vi "manual_control.vi"(0 "Elements+Rates":cluster{"Elements":u16[], "Rates":sgl[]}) -> ()   [LabVIEW 2012]
uses:
  elements.gbl
  number_of_sources.gbl
panel:
  in  "shutdown all":bool
  in  "close":bool
  out "Cluster references":refnum<vi>[][](array[refnum])
  in  "Frame":T1={"Element 1"={"Power (%)"=0.0, "Rate (Å/s)"=0.0, "Gain (Å/s/%)"=0.0, "Set gain"=FALSE, "Manual"=FALSE, "shutdown"=FALSE, "Plot range (min)"=10.0, "Rate graph"=[]}, "Element 2"={"Power (%)"=0.0, "Rate (Å/s)"=0.0, "Gain (Å/s/%)"=0.0, "Set gain"=FALSE, "Manual"=FALSE, "shutdown"=FALSE, "Plot range (min)"=10.0, "Rate graph"=[]}, "Element 3"={"Power (%)"=0.0, "Rate (Å/s)"=0.0, "Gain (Å/s/%)"=0.0, "Set gain"=FALSE, "Manual"=FALSE, "shutdown"=FALSE, "Plot range (min)"=10.0, "Rate graph"=[]}, "Element 4"={"Power (%)"=0.0, "Rate (Å/s)"=0.0, "Gain (Å/s/%)"=0.0, "Set gain"=FALSE, "Manual"=FALSE, "shutdown"=FALSE, "Plot range (min)"=10.0, "Rate graph"=[]}} {"Element 4"."Plot range (min)" min=0.025 step=1.0; "Element 4"."Rate (Å/s)" format="%#.2f"; "Element 4"."Power (%)" min=0 max=90 step=0.1 format="%.2f"; "Element 4"."Gain (Å/s/%)" format="%.1f"; "Element 3"."Plot range (min)" min=0.025 step=1.0; "Element 3"."Rate (Å/s)" format="%#.2f"; "Element 3"."Power (%)" min=0 max=90 step=0.1 format="%.2f"; "Element 3"."Gain (Å/s/%)" format="%.1f"; "Element 2"."Plot range (min)" min=0.025 step=1.0; "Element 2"."Rate (Å/s)" format="%#.2f"; "Element 2"."Power (%)" min=0 max=90 step=0.1 format="%.2f"; "Element 2"."Gain (Å/s/%)" format="%.1f"; "Element 1"."Plot range (min)" min=0.025 step=1.0; "Element 1"."Rate (Å/s)" format="%#.2f"; "Element 1"."Power (%)" min=0 max=90 step=0.1 format="%.2f"; "Element 1"."Gain (Å/s/%)" format="%.1f"}
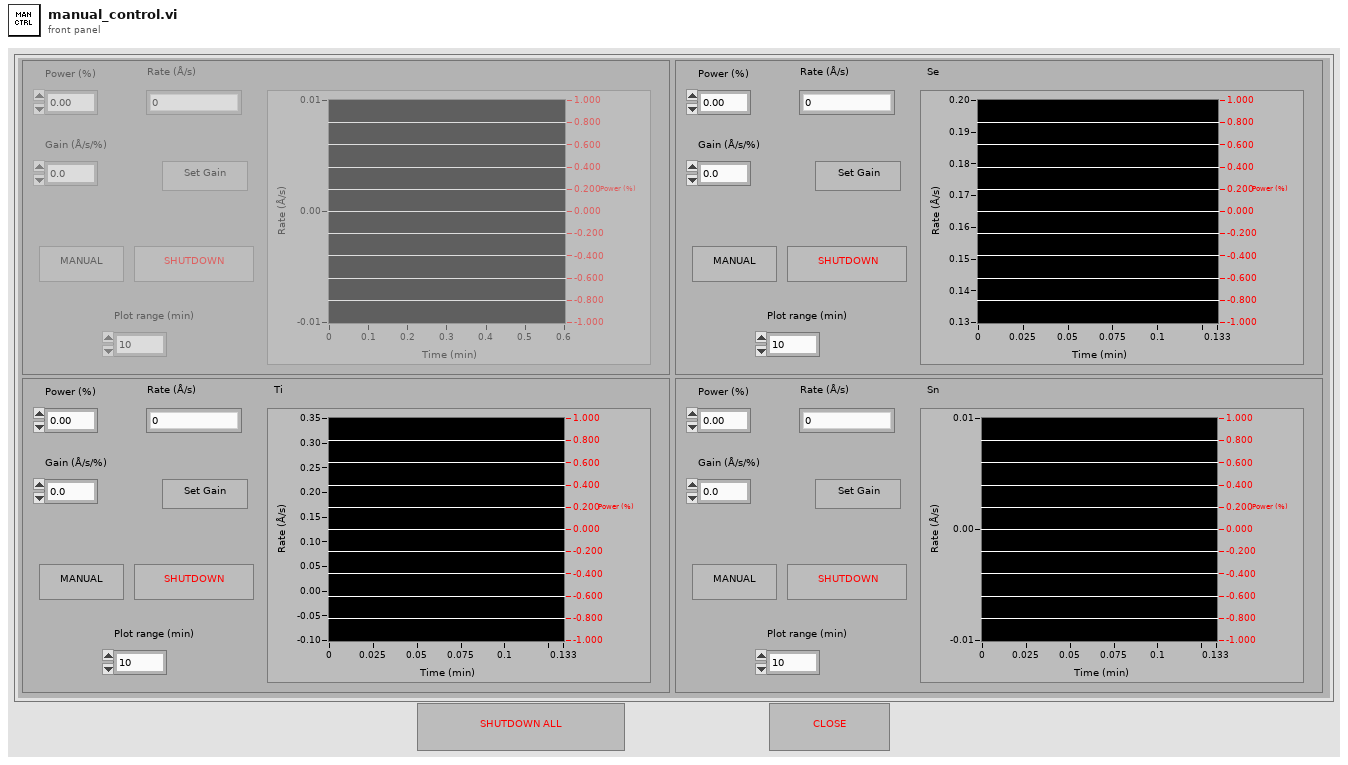
[diagram p1: front panel]
types:
  T1 = cluster{"Element 1":cluster{"Power (%)":sgl, "Rate (Å/s)":sgl, "Gain (Å/s/%)":sgl, "Set gain":bool, "Manual":bool, "shutdown":bool, "Plot range (min)":dbl, "Rate graph":cluster{cluster{sgl, sgl}[]}[]}, "Element 2":cluster{"Power (%)":sgl, "Rate (Å/s)":sgl, "Gain (Å/s/%)":sgl, "Set gain":bool, "Manual":bool, "shutdown":bool, "Plot range (min)":dbl, "Rate graph":cluster{cluster{sgl, sgl}[]}[]}, "Element 3":cluster{"Power (%)":sgl, "Rate (Å/s)":sgl, "Gain (Å/s/%)":sgl, "Set gain":bool, "Manual":bool, "shutdown":bool, "Plot range (min)":dbl, "Rate graph":cluster{cluster{sgl, sgl}[]}[]}, "Element 4":cluster{"Power (%)":sgl, "Rate (Å/s)":sgl, "Gain (Å/s/%)":sgl, "Set gain":bool, "Manual":bool, "shutdown":bool, "Plot range (min)":dbl, "Rate graph":cluster{cluster{sgl, sgl}[]}[]}}
  T2 = enum8{"Enabled", "Disabled", "Disabled and Grayed Out"}
  T3 = cluster{"Element 1":cluster{"Power (%)":bool, "Rate (Å/s)":bool, "Gain (Å/s/%)":bool, "Set gain":bool, "Manual":bool, "shutdown":bool, "Plot range (min)":bool, "Rate graph":cluster{cluster{bool, bool}[]}[]}, "Element 2":cluster{"Power (%)":bool, "Rate (Å/s)":bool, "Gain (Å/s/%)":bool, "Set gain":bool, "Manual":bool, "shutdown":bool, "Plot range (min)":bool, "Rate graph":cluster{cluster{bool, bool}[]}[]}, "Element 3":cluster{"Power (%)":bool, "Rate (Å/s)":bool, "Gain (Å/s/%)":bool, "Set gain":bool, "Manual":bool, "shutdown":bool, "Plot range (min)":bool, "Rate graph":cluster{cluster{bool, bool}[]}[]}, "Element 4":cluster{"Power (%)":bool, "Rate (Å/s)":bool, "Gain (Å/s/%)":bool, "Set gain":bool, "Manual":bool, "shutdown":bool, "Plot range (min)":bool, "Rate graph":cluster{cluster{bool, bool}[]}[]}}
  T4 = cluster{"Power (%)":bool, "Rate (Å/s)":bool, "Gain (Å/s/%)":bool, "Set gain":bool, "Manual":bool, "shutdown":bool, "Plot range (min)":bool, "Rate graph":cluster{cluster{bool, bool}[]}[]}[]
  T5 = cluster{"Power (%)":bool, "Set gain":bool, "Manual":bool, "shutdown":bool}
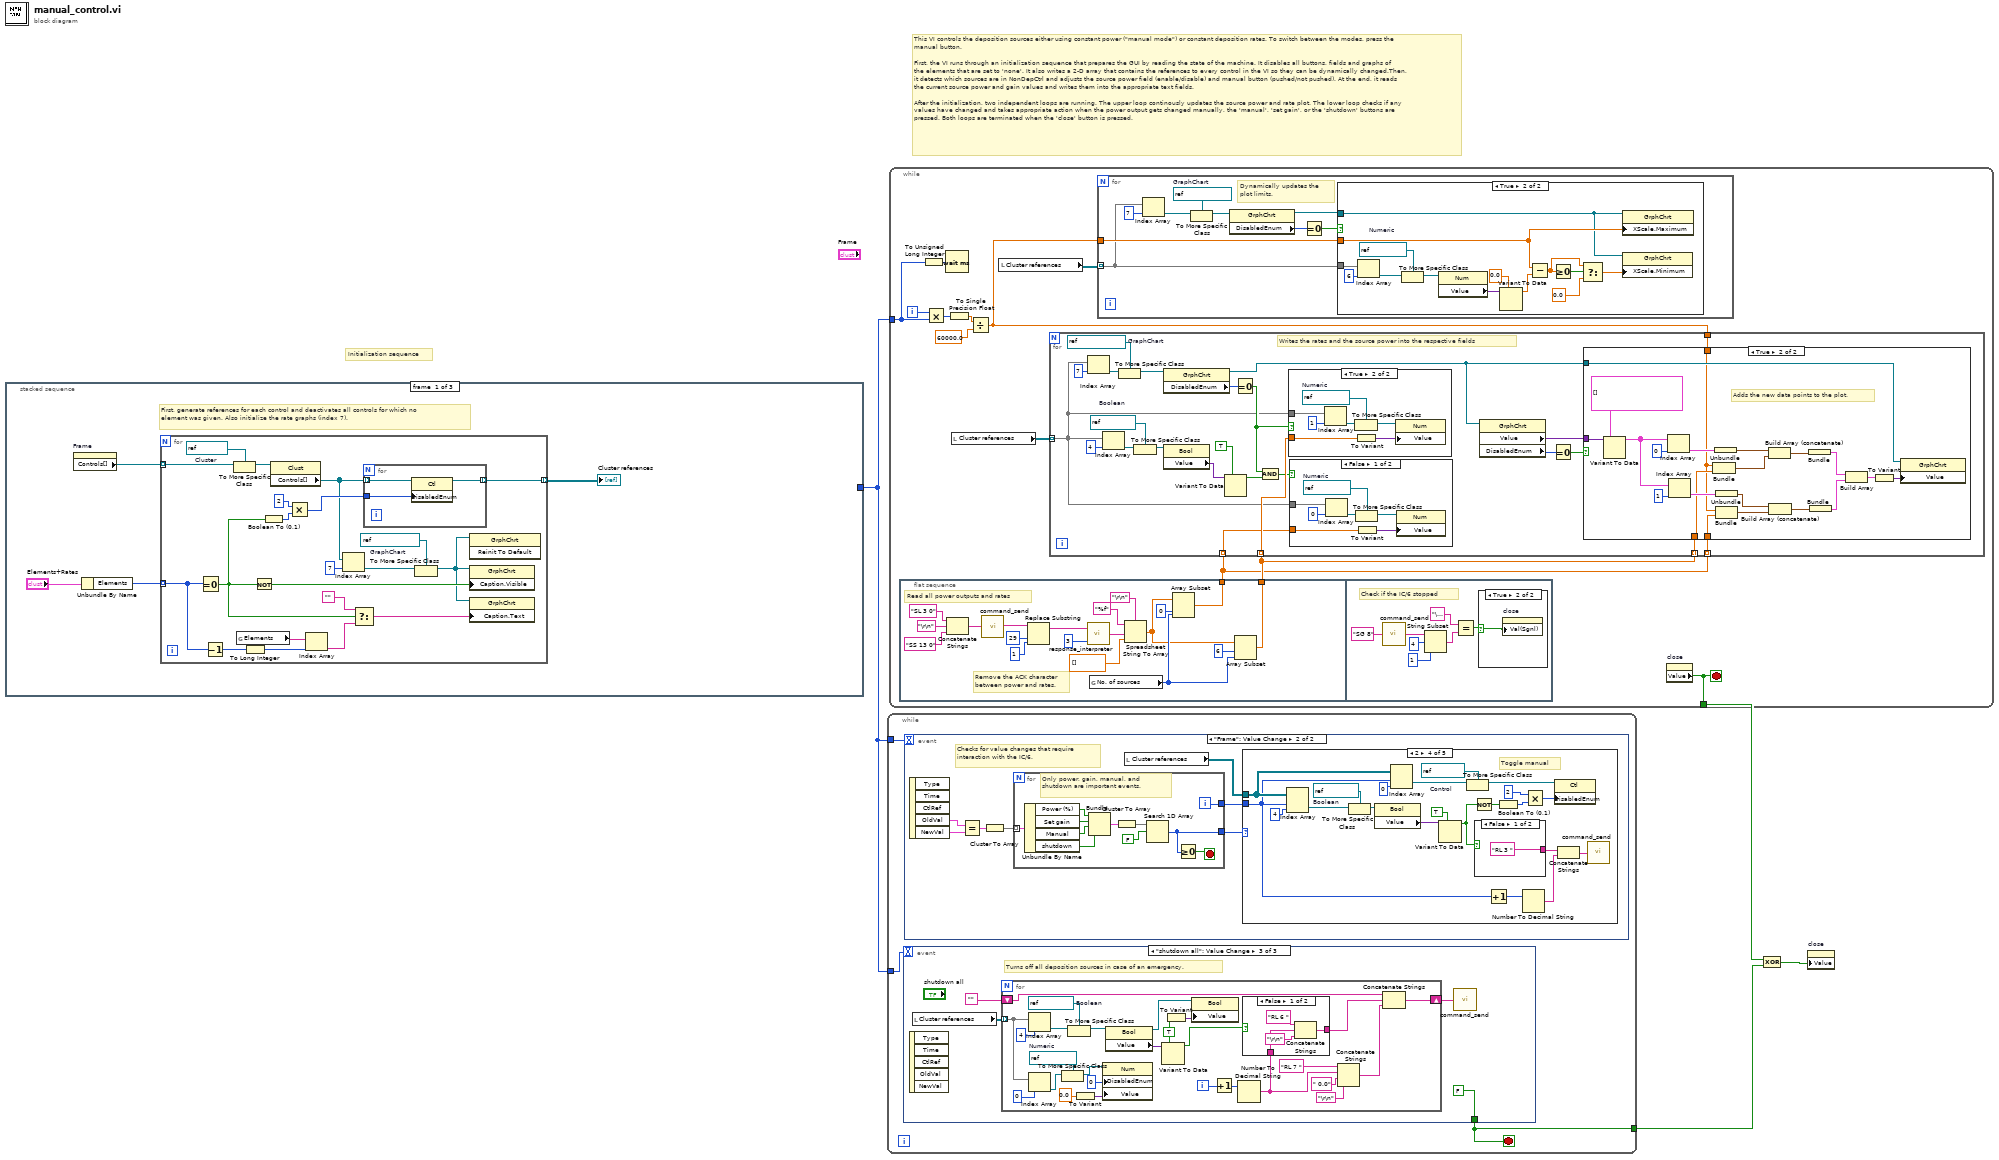
[diagram p0: block diagram]
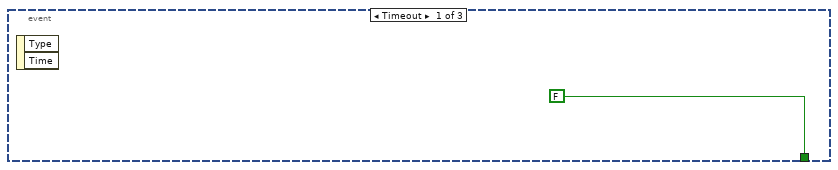
[diagram p2: hidden frame]
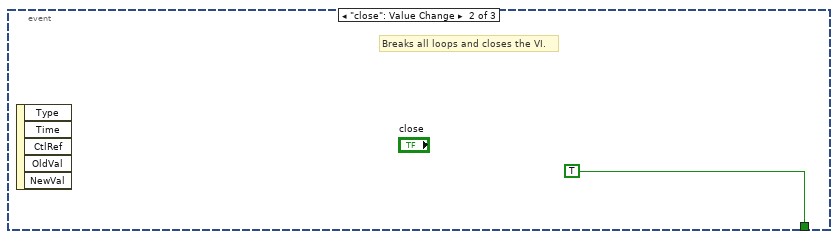
[diagram p3: hidden frame]
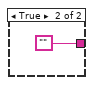
[diagram p4: hidden frame]
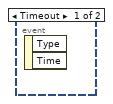
[diagram p5: hidden frame]
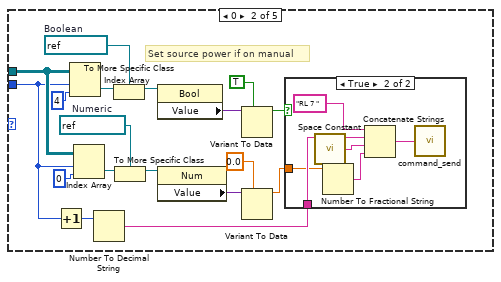
[diagram p7: hidden frame]
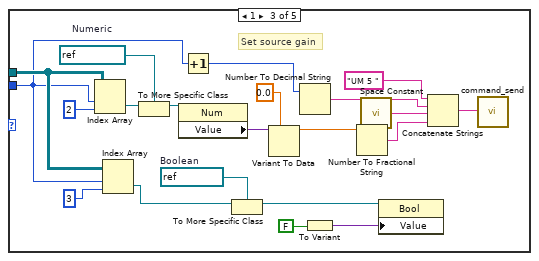
[diagram p9: hidden frame]
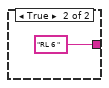
[diagram p10: hidden frame]
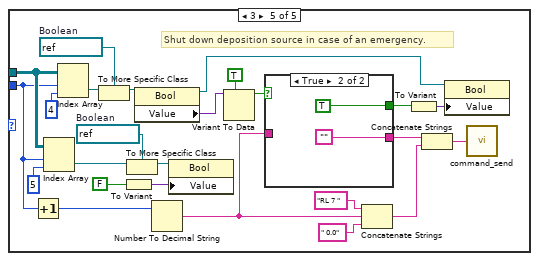
[diagram p11: hidden frame]
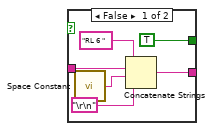
[diagram p12: hidden frame]
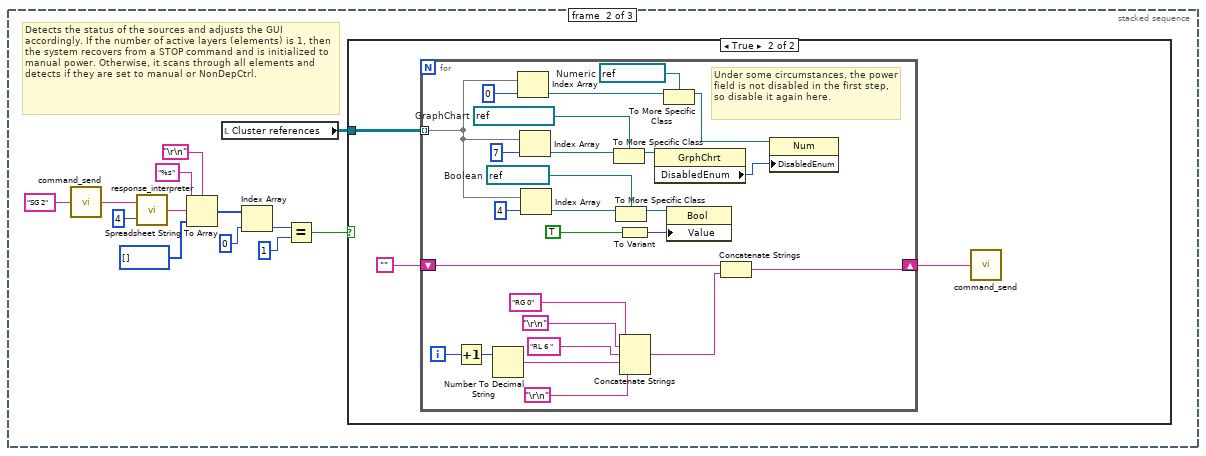
[diagram p18: hidden frame]
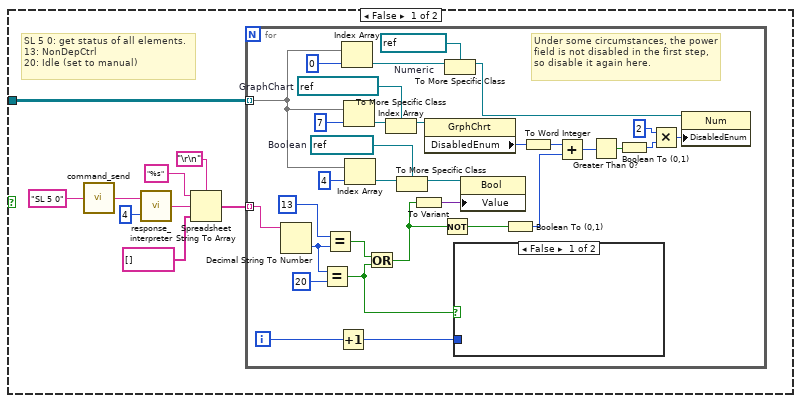
[diagram p19: hidden frame]
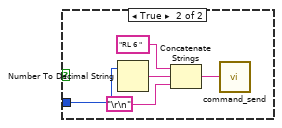
[diagram p20: hidden frame]
diagram:
  # "This VI controls the deposition sources either using constant power (\"manual mode\") or constant deposition rates. To switch between the modes, press the manual button.\n\nFirst, the VI runs through an initialization sequence that prepares the GUI by reading the state of the machine. It disables all buttons, fields and graphs of the elements that are set to 'none'. It also writes a 2-D array that contains the references to every control in the VI so they can be dynamically changed.Then, it detects which sources are in NonDepCtrl and adjusts the source power field (enable/disable) and manual button (pushed/not pushed). At the end, it reads the current source power and gain values and writes them into the appropriate text fields.\n\nAfter the initialization, two independent loops are running. The upper loop continously updates the source power and rate plot. The lower loop checks if any values have changed and takes appropriate action when the power output gets changed manually, the 'manual', 'set gain', or the 'shutdown' buttons are pressed. Both loops are terminated when the 'close' button is pressed."
  # "Initialization sequence"
  n1 = stacked-sequence {
    tunnel: [_ _ 500] -> w4
    frame #0 {
      # "First, generate references for each control and deactivates all controls for which no element was given. Also initialize the rate graphs (index 7)."
      n2 = property on="Frame" class="Clust (strict)"() -> ("Controls[]"=w6:refnum<vi>[])  [unwired: 2 in, 2 out]
      n3 = Unbundle By Name("Elements+Rates") -> ("Elements"=w7:u16[])
      n4 = for {
        tunnel: w7 -> [w13] mode=indexing
        tunnel: w6 -> [w24] mode=indexing
        tunnel: [w23] -> w5 mode=indexing
        w11 = refnum<vi> refnum  # GraphChart
        w26 = refnum<vi> refnum  # Cluster
        n5 = Equal To 0?(x=w13) -> (x = 0?=w15:bool)
        n6 = Decrement(x=w13) -> (x-1=w14:u16)
        n7 = To More Specific Class(target class=w26, reference=w24) -> (specific class reference=w25:refnum<vi>)  [unwired: 1 in, 1 out]
        n8 = global read "elements.gbl" "Elements"() -> (w28:string[])
        n9 = To Long Integer(number=w14) -> (32bit integer=w9:i32)
        n10 = Not(x=w15) -> (.not. x?=w18:bool)
        n11 = Boolean To (0,1)(Boolean=w15) -> (0, 1=w21:i16)
        n12 = property class="Clust"(reference=w25) -> ("Controls[]"=w19:refnum<vi>[])  [unwired: 1 in, 2 out]
        n13 = Multiply(x=i16 2, y=w21) -> (x*y=w20:i16)
        n14 = Index Array(array=w28, index=w9) -> (element=w16:string)
        n15 = Index Array(array=w19, index=7) -> (element=w12:refnum<vi>)
        n16 = Select(t="", s=w15, f=w16) -> (s? t:f=w27:string)
        n17 = for {
          tunnel: w19 -> [w32] mode=indexing
          tunnel: [w31] -> w23 mode=indexing
          tunnel: w20 -> [w30]
          n18 = property class="Ctl"(reference=w32, "DisabledEnum"=w30) -> (reference out=w31:refnum<vi>)  [unwired: 1 in, 1 out]
        }
        n19 = To More Specific Class(target class=w11, reference=w12) -> (specific class reference=w10:refnum<vi>)  [unwired: 1 in, 1 out]
        n20 = invoke class="GrphChrt" method="Reinit To Default"(reference=w10) -> ()  [unwired: 2 in, 3 out]
        n21 = property class="GrphChrt"(reference=w10, "Caption.Visible"=w18) -> ()  [unwired: 1 in, 2 out]
        n22 = property class="GrphChrt"(reference=w10, "Caption.Text"=w27) -> ()  [unwired: 1 in, 2 out]
      }
      "Cluster references" <- w5
    }
    frame #1 {
      # "Detects the status of the sources and adjusts the GUI accordingly. If the number of active layers (elements) is 1, then the system recovers from a STOP command and is initialized to manual power. Otherwise, it scans through all elements and detects if they are set to manual or NonDepCtrl."
      n23 = call "command_send.vi"("Commands"="SG 2") -> ("Response"=w43:string)
      n24 = call "response_interpreter.vi"("Response type"=u16 4, "Response hex"=w43) -> ("Response (readable)"=w42:string)
      n25 = Spreadsheet String To Array(delimiter (Tab)="\r\n", format string="%s", spreadsheet string=w42, array type (2D Dbl)=i32[] []) -> (array=w39:i32[])
      n26 = local read "Cluster references"() -> (w33:refnum<vi>[][])
      n27 = Index Array(array=w39, index=0) -> (element=w36:i32)
      n28 = Equal?(x=w36, y=1) -> (x = y?=w34:bool)
      n29 = case shown="True" w34 {
        tunnel: w33 -> [w46 w94]
        frame False {
          # "SL 5 0: get status of all elements.\n13: NonDepCtrl\n20: Idle (set to manual)"
          n30 = call "command_send.vi"("Commands"="SL 5 0") -> ("Response"=w53:string)
          n31 = call "response_interpreter.vi"("Response type"=u16 4, "Response hex"=w53) -> ("Response (readable)"=w49:string)
          n32 = Spreadsheet String To Array(delimiter (Tab)="\r\n", format string="%s", spreadsheet string=w49, array type (2D Dbl)=string[] []) -> (array=w47:string[])
          n33 = for {
            tunnel: w47 -> [w69] mode=indexing
            tunnel: w46 -> [w73] mode=indexing
            i -> [w65]
            w75 = refnum<vi> refnum  # Numeric
            w80 = refnum<vi> refnum  # Boolean
            w83 = refnum<vi> refnum  # GraphChart
            # "Under some circumstances, the power field is not disabled in the first step, so disable it again here."
            n34 = Decimal String To Number(string=w69) -> (number=w71:i32)  [unwired: 2 in, 1 out]
            n35 = Equal?(x=w71, y=20) -> (x = y?=w67:bool)
            n36 = Equal?(x=13, y=w71) -> (x = y?=w68:bool)
            n37 = Increment(x=w65) -> (x+1=w66:i32)
            n38 = Index Array(array=w73, index=0) -> (element=w76:refnum<vi>)
            n39 = Index Array(array=w73, index=7) -> (element=w85:refnum<vi>)
            n40 = Index Array(array=w73, index=4) -> (element=w81:refnum<vi>)
            n41 = Or(x=w68, y=w67) -> (x .or. y?=w64:bool)
            n42 = To More Specific Class(target class=w83, reference=w85) -> (specific class reference=w84:refnum<vi>)  [unwired: 1 in, 1 out]
            n43 = To More Specific Class(target class=w80, reference=w81) -> (specific class reference=w79:refnum<vi>)  [unwired: 1 in, 1 out]
            n44 = To Variant(anything=w64) -> (Variant=w78:variant)
            n45 = property class="GrphChrt"(reference=w84) -> ("DisabledEnum"=w57:T2)  [unwired: 1 in, 2 out]
            n46 = Not(x=w64) -> (.not. x?=w59:bool)
            n47 = To More Specific Class(target class=w75, reference=w76) -> (specific class reference=w74:refnum<vi>)  [unwired: 1 in, 1 out]
            n48 = case shown="False" w67 {
              tunnel: w66 -> [_ w87]
              frame False {
              }
              frame True {
                n49 = Number To Decimal String(number=w87) -> (decimal integer string=w89:string)  [unwired: 1 in]
                n50 = Concatenate Strings("RL 6 ", w89, "\r\n") -> (w88:string)
                n51 = call "command_send.vi"("Commands"=w88) -> ()  [unwired: 1 out]
              }
            }
            n52 = property class="Bool"(reference=w79, "Value"=w78) -> ()  [unwired: 1 in, 2 out]
            n53 = Boolean To (0,1)(Boolean=w59) -> (0, 1=w56:i16)
            n54 = To Word Integer(number=w57) -> (16bit integer=w55:i16)
            n55 = Add(x=w55, y=w56) -> (x+y=w58:i16)
            n56 = Greater Than 0?(x=w58) -> (x > 0?=w60:bool)
            n57 = Boolean To (0,1)(Boolean=w60) -> (0, 1=w61:i16)
            n58 = Multiply(x=i16 2, y=w61) -> (x*y=w63:i16)
            n59 = property class="Num"(reference=w74, "DisabledEnum"=w63) -> ()  [unwired: 1 in, 2 out]
          }
        }
        frame True {
          n60 = for {
            tunnel: w94 -> [w100] mode=indexing
            shift-right: [w101] -> w92
            shift-left: "" -> [w102]
            i -> [w104]
            w97 = refnum<vi> refnum  # Numeric
            w114 = refnum<vi> refnum  # Boolean
            w117 = refnum<vi> refnum  # GraphChart
            # "Under some circumstances, the power field is not disabled in the first step, so disable it again here."
            n61 = Increment(x=w104) -> (x+1=w105:i32)
            n62 = Number To Decimal String(number=w105) -> (decimal integer string=w110:string)  [unwired: 1 in]
            n63 = Index Array(array=w100, index=0) -> (element=w98:refnum<vi>)
            n64 = Index Array(array=w100, index=7) -> (element=w119:refnum<vi>)
            n65 = Index Array(array=w100, index=4) -> (element=w115:refnum<vi>)
            n66 = To More Specific Class(target class=w117, reference=w119) -> (specific class reference=w118:refnum<vi>)  [unwired: 1 in, 1 out]
            n67 = To More Specific Class(target class=w114, reference=w115) -> (specific class reference=w113:refnum<vi>)  [unwired: 1 in, 1 out]
            n68 = To Variant(anything=TRUE) -> (Variant=w111:variant)
            n69 = Concatenate Strings("RG 0", "\r\n", "RL 6 ", w110, "\r\n") -> (w103:string)
            n70 = property class="GrphChrt"(reference=w118) -> ("DisabledEnum"=w95:T2)  [unwired: 1 in, 2 out]
            n71 = To More Specific Class(target class=w97, reference=w98) -> (specific class reference=w96:refnum<vi>)  [unwired: 1 in, 1 out]
            n72 = property class="Bool"(reference=w113, "Value"=w111) -> ()  [unwired: 1 in, 2 out]
            n73 = Concatenate Strings(w102, w103) -> (w101:string)
            n74 = property class="Num"(reference=w96, "DisabledEnum"=w95) -> ()  [unwired: 1 in, 2 out]
          }
          n75 = call "command_send.vi"("Commands"=w92) -> ()  [unwired: 1 out]
        }
      }
    }
    frame #2 {
      # "At last, read the current power output (SL 3) and the gain (QM 5) for each element, and write them into the appropriate fields."
      n76 = call "command_send.vi"("Commands"="SL 3 0") -> ("Response"=w129:string)
      n77 = local read "Cluster references"() -> (w122:refnum<vi>[][])
      n78 = call "response_interpreter.vi"("Response type"=u16 3, "Response hex"=w129) -> ("Response (readable)"=w125:string)
      n79 = Spreadsheet String To Array(delimiter (Tab)="\r\n", format string="%f", spreadsheet string=w125, array type (2D Dbl)=sgl[] []) -> (array=w123:sgl[])
      n80 = for {
        tunnel: w123 -> [w138] mode=indexing
        tunnel: w122 -> [w137] mode=indexing
        i -> [w151]
        w139 = refnum<vi> refnum  # Numeric
        w141 = refnum<vi> refnum  # Numeric
        n81 = Increment(x=w151) -> (x+1=w150:i32)
        n82 = Number To Decimal String(number=w150) -> (decimal integer string=w149:string)  [unwired: 1 in]
        n83 = Concatenate Strings("QM 5 ", w149) -> (w148:string)
        n84 = call "command_send.vi"("Commands"=w148) -> ("Response"=w147:string)
        n85 = Index Array(array=w137, index=0) -> (element=w143:refnum<vi>)
        n86 = Index Array(array=w137, index=2) -> (element=w136:refnum<vi>)
        n87 = call "response_interpreter.vi"("Response type"=u16 3, "Response hex"=w147) -> ("Response (readable)"=w132:string)
        n88 = To Variant(anything=w138) -> (Variant=w140:variant)
        n89 = To More Specific Class(target class=w141, reference=w143) -> (specific class reference=w142:refnum<vi>)  [unwired: 1 in, 1 out]
        n90 = To More Specific Class(target class=w139, reference=w136) -> (specific class reference=w135:refnum<vi>)  [unwired: 1 in, 1 out]
        n91 = Fract/Exp String To Number(string=w132, default (0 dbl)=sgl 0.0) -> (number=w131:sgl)  [unwired: 2 in, 1 out]
        n92 = property class="Num"(reference=w142, "Value"=w140) -> ()  [unwired: 1 in, 2 out]
        n93 = To Variant(anything=w131) -> (Variant=w134:variant)
        n94 = property class="Num"(reference=w135, "Value"=w134) -> ()  [unwired: 1 in, 2 out]
      }
    }
  }
  n95 = while {
    tunnel: w4 -> [w155]
    tunnel: w4 -> [w154]
    tunnel: [w153] -> w3
    stop <- w153 stop-if-true
    n96 = event shown="[2] \"shutdown all\": Value Change" {
      selector: _ -> [_ _ _]
      dyn-events: _ -> [_ _ _]
      timeout: w154 -> [_ _ _]
      tunnel: [FALSE TRUE FALSE] -> w153
      event Timeout {
        n97 = event-data() -> ()  [unwired: 1 in, 2 out]
      }
      event "close": Value Change {
        # "Breaks all loops and closes the VI."
        n98 = event-data() -> ()  [unwired: 1 in, 5 out]
      }
      event "shutdown all": Value Change {
        # "Turns off all deposition sources in case of an emergency."
        n99 = event-data() -> ()  [unwired: 1 in, 5 out]
        n100 = local read "Cluster references"() -> (w160:refnum<vi>[][])
        n101 = for {
          tunnel: w160 -> [w175] mode=indexing
          shift-right: [w187] -> w158
          shift-left: "" -> [w188]
          i -> [w179]
          w169 = TRUE
          w167 = refnum<vi> refnum  # Numeric
          w177 = refnum<vi> refnum  # Boolean
          n102 = Index Array(array=w175, index=4) -> (element=w178:refnum<vi>)
          n103 = Index Array(array=w175, index=0) -> (element=w166:refnum<vi>)
          n104 = To More Specific Class(target class=w167, reference=w166) -> (specific class reference=w165:refnum<vi>)  [unwired: 1 in, 1 out]
          n105 = To More Specific Class(target class=w177, reference=w178) -> (specific class reference=w173:refnum<vi>)  [unwired: 1 in, 1 out]
          n106 = To Variant(anything=0.0) -> (Variant=w163:variant)
          n107 = property class="Num"(reference=w165, "DisabledEnum"=0, "Value"=w163) -> ()  [unwired: 1 in, 2 out]
          n108 = property class="Bool"(reference=w173) -> (reference out=w168:refnum<vi>, "Value"=w172:variant)  [unwired: 1 in, 1 out]
          n109 = Variant To Data(type=w169, Variant=w172) -> (data=w171:bool)  [unwired: 1 in, 1 out]
          n110 = To Variant(anything=w169) -> (Variant=w170:variant)
          n111 = property class="Bool"(reference=w168, "Value"=w170) -> ()  [unwired: 1 in, 2 out]
          n112 = Increment(x=w179) -> (x+1=w182:i32)
          n113 = Number To Decimal String(number=w182) -> (decimal integer string=w180:string)  [unwired: 1 in]
          n114 = case shown="False" w171 {
            tunnel: [w190 ""] -> w186
            tunnel: w180 -> [w189 _]
            frame False {
              n115 = Concatenate Strings("RL 6 ", w189, "\r\n") -> (w190:string)
            }
            frame True {
            }
          }
          n116 = Concatenate Strings("RL 7 ", w180, " 0.0", "\r\n") -> (w181:string)
          n117 = Concatenate Strings(w188, w186, w181) -> (w187:string)
        }
        n118 = call "command_send.vi"("Commands"=w158) -> ()  [unwired: 1 out]
      }
    }
    n119 = event shown="[1] \"Frame\": Value Change" {
      selector: _ -> [_ _]
      dyn-events: _ -> [_ _]
      timeout: w155 -> [_ _]
      event Timeout {
        n120 = event-data() -> ()  [unwired: 1 in, 2 out]
      }
      event "Frame": Value Change {
        # "Checks for value changes that require interaction with the IC/6."
        n121 = event-data() -> ("OldVal"=w200:T1, "NewVal"=w199:T1)  [unwired: 1 in, 3 out]
        n122 = Equal?(x=w200, y=w199) -> (x = y?=w198:T3)
        n123 = Cluster To Array(cluster=w198) -> (array=w197:T4)
        n124 = for {
          tunnel: w197 -> [w312] mode=indexing
          tunnel: [w304] -> w196
          tunnel: [w302] -> w194
          i -> [w302]
          stop <- w305 stop-if-true
          # "Only power, gain, manual, and shutdown are important events."
          n125 = Unbundle By Name(w312) -> ("Power (%)"=w311:bool, "Set gain"=w310:bool, "Manual"=w309:bool, "shutdown"=w308:bool)
          n126 = Bundle("Power (%)"=w311, "Set gain"=w310, "Manual"=w309, "shutdown"=w308) -> (w307:T5)  [unwired: 1 in]
          n127 = Cluster To Array(cluster=w307) -> (array=w306:bool[])
          n128 = Search 1D Array(1D array=w306, element=FALSE) -> (index of element=w304:i32)  [unwired: 1 in]
          n129 = Greater Or Equal To 0?(x=w304) -> (x >= 0?=w305:bool)
        }
        n130 = local read "Cluster references"() -> (w195:refnum<vi>[][])
        n131 = case shown="2" w196 {
          tunnel: w195 -> [_ w214 w232 w248 w271]
          tunnel: w194 -> [_ w203 w231 w247 w270]
          frame -1, Default {
          }
          frame 0 {
            w218 = refnum<vi> refnum  # Numeric
            w217 = refnum<vi> refnum  # Boolean
            # "Set source power if on manual"
            n132 = Increment(x=w203) -> (x+1=w202:i32)
            n133 = Index Array(array=w214, index (row)=w203, index (col)=4) -> (element=w216:refnum<vi>)
            n134 = Index Array(array=w214, index (row)=w203, index (col)=0) -> (element=w215:refnum<vi>)
            n135 = Number To Decimal String(number=w202) -> (decimal integer string=w201:string)  [unwired: 1 in]
            n136 = To More Specific Class(target class=w217, reference=w216) -> (specific class reference=w211:refnum<vi>)  [unwired: 1 in, 1 out]
            n137 = To More Specific Class(target class=w218, reference=w215) -> (specific class reference=w210:refnum<vi>)  [unwired: 1 in, 1 out]
            n138 = property class="Bool"(reference=w211) -> ("Value"=w209:variant)  [unwired: 1 in, 2 out]
            n139 = property class="Num"(reference=w210) -> ("Value"=w208:variant)  [unwired: 1 in, 2 out]
            n140 = Variant To Data(type=TRUE, Variant=w209) -> (data=w205:bool)  [unwired: 1 in, 1 out]
            n141 = Variant To Data(type=sgl 0.0, Variant=w208) -> (data=w204:sgl)  [unwired: 1 in, 1 out]
            n142 = case shown="True" w205 {
              tunnel: w204 -> [_ w219]
              tunnel: w201 -> [_ w220]
              frame False {
              }
              frame True {
                n143 = call <vilib>:"Space Constant.vi"() -> ("String"=w221:string)
                n144 = Number To Fractional String(number=w219) -> (F-format string=w224:string)  [unwired: 3 in]
                n145 = Concatenate Strings("RL 7 ", w220, w221, w224) -> (w223:string)
                n146 = call "command_send.vi"("Commands"=w223) -> ()  [unwired: 1 out]
              }
            }
          }
          frame 1 {
            w226 = refnum<vi> refnum  # Boolean
            w242 = refnum<vi> refnum  # Numeric
            # "Set source gain"
            n147 = Index Array(array=w232, index (row)=w231, index (col)=2) -> (element=w241:refnum<vi>)
            n148 = Index Array(array=w232, index (row)=w231, index (col)=3) -> (element=w229:refnum<vi>)
            n149 = To More Specific Class(target class=w242, reference=w241) -> (specific class reference=w240:refnum<vi>)  [unwired: 1 in, 1 out]
            n150 = property class="Num"(reference=w240) -> ("Value"=w239:variant)  [unwired: 1 in, 2 out]
            n151 = Increment(x=w231) -> (x+1=w233:i32)
            n152 = To More Specific Class(target class=w226, reference=w229) -> (specific class reference=w228:refnum<vi>)  [unwired: 1 in, 1 out]
            n153 = Variant To Data(type=sgl 0.0, Variant=w239) -> (data=w237:sgl)  [unwired: 1 in, 1 out]
            n154 = Number To Decimal String(number=w233) -> (decimal integer string=w234:string)  [unwired: 1 in]
            n155 = To Variant(anything=FALSE) -> (Variant=w225:variant)
            n156 = Number To Fractional String(number=w237) -> (F-format string=w245:string)  [unwired: 3 in]
            n157 = call <vilib>:"Space Constant.vi"() -> ("String"=w235:string)
            n158 = property class="Bool"(reference=w228, "Value"=w225) -> ()  [unwired: 1 in, 2 out]
            n159 = Concatenate Strings("UM 5 ", w234, w235, w245) -> (w244:string)
            n160 = call "command_send.vi"("Commands"=w244) -> ()  [unwired: 1 out]
          }
          frame 2 {
            w250 = refnum<vi> refnum  # Control
            w264 = refnum<vi> refnum  # Boolean
            # "Toggle manual"
            n161 = Index Array(array=w248, index (row)=w247, index (col)=4) -> (element=w265:refnum<vi>)
            n162 = To More Specific Class(target class=w264, reference=w265) -> (specific class reference=w263:refnum<vi>)  [unwired: 1 in, 1 out]
            n163 = property class="Bool"(reference=w263) -> ("Value"=w262:variant)  [unwired: 1 in, 2 out]
            n164 = Index Array(array=w248, index (row)=w247, index (col)=0) -> (element=w252:refnum<vi>)
            n165 = Variant To Data(type=TRUE, Variant=w262) -> (data=w257:bool)  [unwired: 1 in, 1 out]
            n166 = To More Specific Class(target class=w250, reference=w252) -> (specific class reference=w251:refnum<vi>)  [unwired: 1 in, 1 out]
            n167 = Not(x=w257) -> (.not. x?=w258:bool)
            n168 = case shown="False" w257 {
              tunnel: ["RL 3 " "RL 6 "] -> w259
              frame False {
              }
              frame True {
              }
            }
            n169 = Increment(x=w247) -> (x+1=w260:i32)
            n170 = Boolean To (0,1)(Boolean=w258) -> (0, 1=w256:i16)
            n171 = Number To Decimal String(number=w260) -> (decimal integer string=w255:string)  [unwired: 1 in]
            n172 = Multiply(x=i16 2, y=w256) -> (x*y=w249:i16)
            n173 = property class="Ctl"(reference=w251, "DisabledEnum"=w249) -> ()  [unwired: 1 in, 2 out]
            n174 = Concatenate Strings(w259, w255) -> (w246:string)
            n175 = call "command_send.vi"("Commands"=w246) -> ()  [unwired: 1 out]
          }
          frame 3 {
            w276 = refnum<vi> refnum  # Boolean
            w281 = refnum<vi> refnum  # Boolean
            # "Shut down deposition source in case of an emergency."
            n176 = Increment(x=w270) -> (x+1=w293:i32)
            n177 = Index Array(array=w271, index (row)=w270, index (col)=5) -> (element=w272:refnum<vi>)
            n178 = Index Array(array=w271, index (row)=w270, index (col)=4) -> (element=w282:refnum<vi>)
            n179 = To More Specific Class(target class=w281, reference=w282) -> (specific class reference=w280:refnum<vi>)  [unwired: 1 in, 1 out]
            n180 = To Variant(anything=FALSE) -> (Variant=w274:variant)
            n181 = To More Specific Class(target class=w276, reference=w272) -> (specific class reference=w275:refnum<vi>)  [unwired: 1 in, 1 out]
            n182 = property class="Bool"(reference=w280) -> (reference out=w278:refnum<vi>, "Value"=w279:variant)  [unwired: 1 in, 1 out]
            n183 = Number To Decimal String(number=w293) -> (decimal integer string=w290:string)  [unwired: 1 in]
            n184 = property class="Bool"(reference=w275, "Value"=w274) -> ()  [unwired: 1 in, 2 out]
            n185 = Variant To Data(type=TRUE, Variant=w279) -> (data=w285:bool)  [unwired: 1 in, 1 out]
            n186 = case shown="True" w285 {
              tunnel: [w299 ""] -> w289
              tunnel: w290 -> [w295 _]
              tunnel: [TRUE TRUE] -> w286
              frame False {
                n187 = call <vilib>:"Space Constant.vi"() -> ("String"=w296:string)
                n188 = Concatenate Strings("RL 6 ", w295, w296, "\r\n") -> (w299:string)
              }
              frame True {
              }
            }
            n189 = Concatenate Strings("RL 7 ", w290, " 0.0") -> (w288:string)
            n190 = To Variant(anything=w286) -> (Variant=w277:variant)
            n191 = Concatenate Strings(w289, w288) -> (w287:string)
            n192 = property class="Bool"(reference=w278, "Value"=w277) -> ()  [unwired: 1 in, 2 out]
            n193 = call "command_send.vi"("Commands"=w287) -> ()  [unwired: 1 out]
          }
        }
      }
    }
  }
  n194 = while {
    tunnel: w4 -> [w323]
    tunnel: [w317] -> w2
    i -> [w324]
    stop <- w317 stop-if-true
    n195 = flat-sequence {
      tunnel: [w415] -> w315
      tunnel: [w414] -> w316
      frame #0 {
        # "Remove the ACK character between power and rates."
        # "Read all power outputs and rates"
        n196 = Concatenate Strings("SL 3 0", "\r\n", "SS 13 0") -> (w420:string)
        n197 = call "command_send.vi"("Commands"=w420) -> ("Response"=w407:string)
        n198 = Replace Substring(2:1, 3:29, 5:w407) -> (1:w410:string)  [unwired: 1 in, 1 out]
        n199 = call "response_interpreter.vi"("Response type"=u16 3, "Response hex"=w410) -> ("Response (readable)"=w423:string)
        n200 = global read "number_of_sources.gbl" "No. of sources"() -> (w412:i32)
        n201 = Spreadsheet String To Array(delimiter (Tab)="\r\n", format string="%f", spreadsheet string=w423, array type (2D Dbl)=sgl[] []) -> (array=w411:sgl[])
        n202 = Array Subset(array=w411, index=0, length=w412) -> (w415:sgl[])
        n203 = Array Subset(array=w411, index=6, length=w412) -> (w414:sgl[])
      }
      frame #1 {
        # "Check if the IC/6 stopped"
        n204 = call "command_send.vi"("Commands"="SG 8") -> ("Response"=w431:string)
        n205 = String Subset(string=w431, offset (0)=4, length (rest)=1) -> (substring=w427:string)
        n206 = Equal?(x="\u0006", y=w427) -> (x = y?=w426:bool)
        n207 = case shown="True" w426 {
          selector: w426 -> [_ w433]
          frame False {
          }
          frame True {
            n208 = property on="close" class="Bool (strict)"("Val(Sgnl)"=w433) -> ()  [unwired: 2 in, 2 out]
          }
        }
      }
    }
    n209 = To Unsigned Long Integer(number=w323) -> (unsigned 32bit integer=w314:u32)
    n210 = Multiply(x=w324, y=w323) -> (x*y=w322:i32)
    n211 = Wait (ms)(milliseconds to wait=w314) -> ()  [unwired: 1 out]
    n212 = To Single Precision Float(number=w322) -> (single precision float=w313:sgl)
    n213 = local read "Cluster references"() -> (w319:refnum<vi>[][])
    n214 = Divide(x=w313, y=sgl 60000.0) -> (x/y=w318:sgl)
    n215 = local read "Cluster references"() -> (w320:refnum<vi>[][])
    n216 = for {
      tunnel: w319 -> [w330] mode=indexing
      tunnel: w315 -> [w329] mode=indexing
      tunnel: w316 -> [w332] mode=indexing
      tunnel: w318 -> [w328]
      tunnel: w315 -> [w327] mode=indexing
      tunnel: w316 -> [w326] mode=indexing
      w342 = refnum<vi> refnum  # Boolean
      w347 = refnum<vi> refnum  # GraphChart
      # "Writes the rates and the source power into the respective fields"
      n217 = Index Array(array=w330, index=7) -> (element=w346:refnum<vi>)
      n218 = Index Array(array=w330, index=4) -> (element=w341:refnum<vi>)
      n219 = To More Specific Class(target class=w347, reference=w346) -> (specific class reference=w337:refnum<vi>)  [unwired: 1 in, 1 out]
      n220 = To More Specific Class(target class=w342, reference=w341) -> (specific class reference=w340:refnum<vi>)  [unwired: 1 in, 1 out]
      n221 = property class="Bool"(reference=w340) -> ("Value"=w339:variant)  [unwired: 1 in, 2 out]
      n222 = property class="GrphChrt"(reference=w337) -> (reference out=w325:refnum<vi>, "DisabledEnum"=w345:T2)  [unwired: 1 in, 1 out]
      n223 = Variant To Data(type=TRUE, Variant=w339) -> (data=w338:bool)  [unwired: 1 in, 1 out]
      n224 = Equal To 0?(x=w345) -> (x = 0?=w333:bool)
      n225 = And(x=w333, y=w338) -> (x .and. y?=w331:bool)
      n226 = case shown="True" w333 {
        tunnel: w330 -> [_ w352]
        tunnel: w332 -> [_ w349]
        frame False {
        }
        frame True {
          w355 = refnum<vi> refnum  # Numeric
          n227 = Index Array(array=w352, index=1) -> (element=w354:refnum<vi>)
          n228 = To More Specific Class(target class=w355, reference=w354) -> (specific class reference=w351:refnum<vi>)  [unwired: 1 in, 1 out]
          n229 = To Variant(anything=w349) -> (Variant=w350:variant)
          n230 = property class="Num"(reference=w351, "Value"=w350) -> ()  [unwired: 1 in, 2 out]
        }
      }
      n231 = case shown="False" w331 {
        tunnel: w330 -> [w380 _]
        tunnel: w329 -> [w377 _]
        frame False {
          w383 = refnum<vi> refnum  # Numeric
          n232 = Index Array(array=w380, index=0) -> (element=w382:refnum<vi>)
          n233 = To More Specific Class(target class=w383, reference=w382) -> (specific class reference=w379:refnum<vi>)  [unwired: 1 in, 1 out]
          n234 = To Variant(anything=w377) -> (Variant=w378:variant)
          n235 = property class="Num"(reference=w379, "Value"=w378) -> ()  [unwired: 1 in, 2 out]
        }
        frame True {
        }
      }
      n236 = property class="GrphChrt"(reference=w325) -> ("Value"=w334:variant, "DisabledEnum"=w336:T2)  [unwired: 1 in, 2 out]
      n237 = Equal To 0?(x=w336) -> (x = 0?=w335:bool)
      n238 = case shown="True" w335 {
        tunnel: w334 -> [_ w375]
        tunnel: w328 -> [_ w357]
        tunnel: w327 -> [_ w376]
        tunnel: w326 -> [_ w363]
        tunnel: w325 -> [_ w360]
        frame False {
        }
        frame True {
          # "Adds the new data points to the plot."
          n239 = Variant To Data(type=cluster{cluster{sgl, sgl}[]}[] [], Variant=w375) -> (data=w367:cluster{cluster{sgl, sgl}[]}[])  [unwired: 1 in, 1 out]
          n240 = Index Array(array=w367, index=0) -> (element=w372:cluster{cluster{sgl, sgl}[]})
          n241 = Index Array(array=w367, index=1) -> (element=w366:cluster{cluster{sgl, sgl}[]})
          n242 = Bundle(w357, w363) -> (w370:cluster{sgl, sgl})  [unwired: 1 in]
          n243 = Unbundle(w372) -> (w371:cluster{sgl, sgl}[])
          n244 = Unbundle(w366) -> (w364:cluster{sgl, sgl}[])
          n245 = Bundle(w357, w376) -> (w365:cluster{sgl, sgl})  [unwired: 1 in]
          n246 = Build Array (concatenate)(w371, w370) -> (w373:cluster{sgl, sgl}[])
          n247 = Build Array (concatenate)(w364, w365) -> (w362:cluster{sgl, sgl}[])
          n248 = Bundle(w373) -> (w374:cluster{cluster{sgl, sgl}[]})  [unwired: 1 in]
          n249 = Bundle(w362) -> (w361:cluster{cluster{sgl, sgl}[]})  [unwired: 1 in]
          n250 = Build Array(w374, w361) -> (w358:cluster{cluster{sgl, sgl}[]}[])
          n251 = To Variant(anything=w358) -> (Variant=w359:variant)
          n252 = property class="GrphChrt"(reference=w360, "Value"=w359) -> ()  [unwired: 1 in, 2 out]
        }
      }
    }
    n253 = for {
      tunnel: w320 -> [w388] mode=indexing
      tunnel: w318 -> [w389]
      w391 = refnum<vi> refnum  # GraphChart
      # "Dynamically updates the plot limits."
      n254 = Index Array(array=w388, index=7) -> (element=w390:refnum<vi>)
      n255 = To More Specific Class(target class=w391, reference=w390) -> (specific class reference=w387:refnum<vi>)  [unwired: 1 in, 1 out]
      n256 = property class="GrphChrt"(reference=w387) -> (reference out=w386:refnum<vi>, "DisabledEnum"=w385:T2)  [unwired: 1 in, 1 out]
      n257 = Equal To 0?(x=w385) -> (x = 0?=w384:bool)
      n258 = case shown="True" w384 {
        tunnel: w389 -> [_ w395]
        tunnel: w386 -> [_ w394]
        tunnel: w388 -> [_ w393]
        frame False {
        }
        frame True {
          w404 = refnum<vi> refnum  # Numeric
          n259 = Index Array(array=w393, index=6) -> (element=w405:refnum<vi>)
          n260 = To More Specific Class(target class=w404, reference=w405) -> (specific class reference=w403:refnum<vi>)  [unwired: 1 in, 1 out]
          n261 = property class="Num"(reference=w403) -> ("Value"=w402:variant)  [unwired: 1 in, 2 out]
          n262 = Variant To Data(type=sgl 0.0, Variant=w402) -> (data=w400:sgl)  [unwired: 1 in, 1 out]
          n263 = Subtract(x=w395, y=w400) -> (x-y=w396:sgl)
          n264 = Greater Or Equal To 0?(x=w396) -> (x >= 0?=w398:bool)
          n265 = Select(t=w396, s=w398, f=sgl 0.0) -> (s? t:f=w397:sgl)
          n266 = property class="GrphChrt"(reference=w394, "XScale.Maximum"=w395) -> ()  [unwired: 1 in, 2 out]
          n267 = property class="GrphChrt"(reference=w394, "XScale.Minimum"=w397) -> ()  [unwired: 1 in, 2 out]
        }
      }
    }
    n268 = property on="close" class="Bool (strict)"() -> ("Value"=w317:bool)  [unwired: 2 in, 2 out]
  }
  n269 = Exclusive Or(1:w3, 2:w2) -> (0:w1:bool)
  n270 = property on="close" class="Bool (strict)"("Value"=w1) -> ()  [unwired: 2 in, 2 out]
